vi "TDMS.GetCycledChannels.vi"(8 "error in (no error)":errorcluster, 11 "TDMS Ref":refnum<k34>) -> (0 "error out":errorcluster, 1 "DUTs":string[](array[string]), 2 "Cycled":bool[](array[boolean]), 3 "TDMS Ref":refnum<k34>)   [LabVIEW 2015, in "TestStand Analysis Steps.lvlib"]
uses:
  TestStand Analysis Steps.lvlib
  Shared/Constants.vi
  Shared/Shared.lvlib
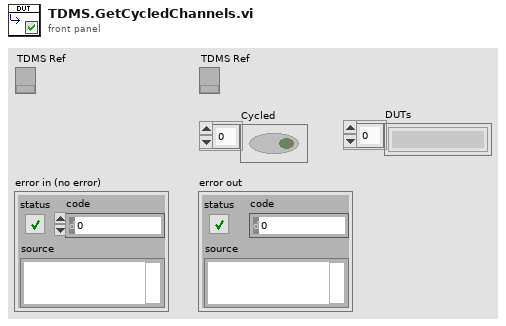
[diagram p1: front panel]
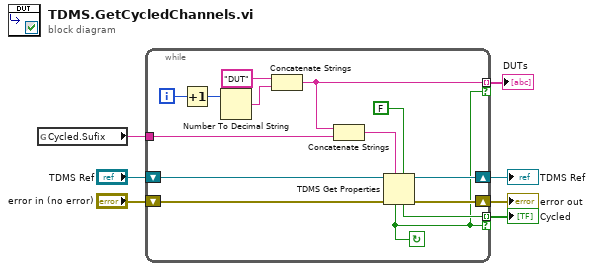
[diagram p0: block diagram]
diagram:
  n1 = global read "Constants.vi" "Cycled.Sufix"() -> (w1:string)
  n2 = while {
    shift-right: [w20] -> w4
    shift-left: "error in (no error)" -> [w21]
    shift-right: [w18] -> w6
    shift-left: "TDMS Ref" -> [w19]
    tunnel: [w15] -> w7 mode=indexing if=w8
    tunnel: w1 -> [w14]
    tunnel: [w9] -> w2 mode=indexing if=w8
    i -> [w13]
    stop <- w8 continue-if-true
    n3 = Increment(x=w13) -> (x+1=w12:i32)
    n4 = Number To Decimal String(number=w12) -> (decimal integer string=w10:string)  [unwired: 1 in]
    n5 = Concatenate Strings("DUT", w10) -> (w9:string)
    n6 = Concatenate Strings(w9, w14) -> (w17:string)
    n7 = TDMS Get Properties(5:FALSE, 7:w17, 8:w21, 11:w19) -> (0:w20:errorcluster, 3:w18:refnum<k34>, 4:w15:bool, 6:w8:bool)  [unwired: 2 in, 2 out]
  }
  "Cycled" <- w7
  "TDMS Ref" <- w6
  "error out" <- w4
  "DUTs" <- w2
